vi "Dispose.vi"(8 "error in (no error)":errorcluster, 11 "PalmSens in":refnum<class "PalmSens.lvclass">) -> (0 "error out":errorcluster, 3 "PalmSens out":refnum<class "PalmSens.lvclass">)   [LabVIEW 2025, in "PalmSens.lvclass"]
uses:
  PalmSens.lvclass
  PalmSens.lvclass/PalmSens.ctl
  C:/Users/stef/code/palmsenssdk/labview/PalmSens/Libraries/PalmSens.Core.Simplified.LabVIEW.dll
  Libraries/PalmSens.Core.Simplified.LabVIEW.dll
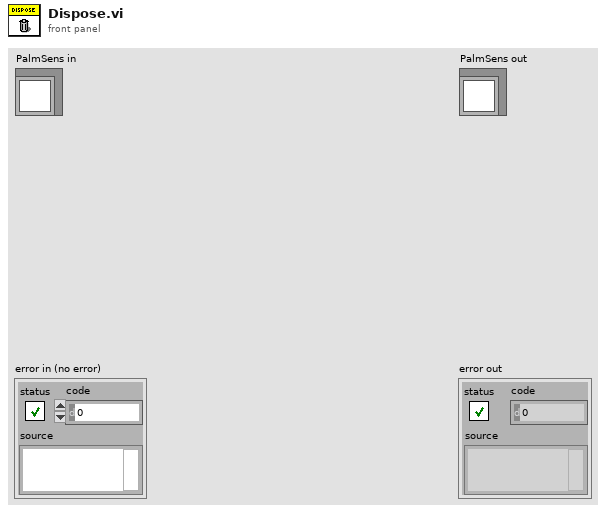
[diagram p1: front panel]
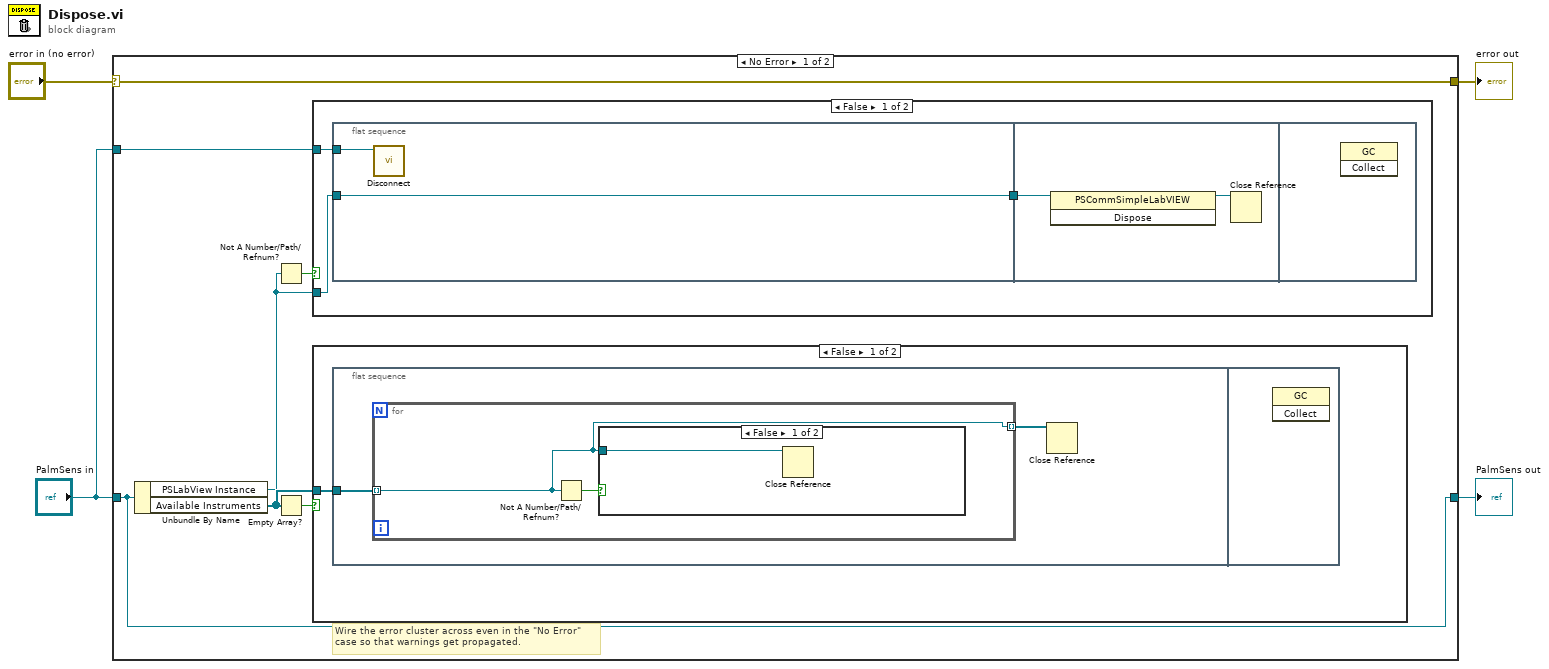
[diagram p0: block diagram]
diagram:
  n1 = case shown="No Error" "error in (no error)" {
    selector: "error in (no error)" -> [w11 w26]
    tunnel: [w11 w26] -> w3
    tunnel: [w10 w25] -> w2
    tunnel: "PalmSens in" -> [w10 w25]
    tunnel: "PalmSens in" -> [w5 _]
    frame No Error {
      # "Wire the error cluster across even in the \"No Error\"\ncase so that warnings get propagated."
      n2 = Unbundle By Name(w10) -> ("PSLabView Instance"=w6:refnum<k24>, "Available Instruments"=w8:refnum<k24>[])
      n3 = Not A Number/Path/Refnum?(number/path/refnum=w6) -> (NaN/Path/Refnum?=w7:bool)
      n4 = Empty Array?(array=w8) -> (empty?=w9:bool)
      n5 = case shown="False" w7 {
        tunnel: w6 -> [w14 _]
        tunnel: w5 -> [w12 _]
        frame False {
          n6 = flat-sequence {
            tunnel: w14 -> [w15]
            tunnel: [w15] -> w13
            tunnel: w12 -> [w16]
            tunnel: w13 -> [w18]
            frame #0 {
              n7 = call-dynamic "Disconnect.vi"("PalmSens in"=w16) -> ()  [unwired: 9 in, 2 out]
            }
            frame #1 {
              n8 = invoke class="PSCommSimpleLabVIEW" method="Dispose"(reference=w18) -> (reference out=w17:refnum<k24>)  [unwired: 2 in, 2 out]
              n9 = Close Reference(reference=w17) -> ()  [unwired: 1 in, 1 out]
            }
            frame #2 {
              n10 = invoke class="GC" method="Collect"() -> ()  [unwired: 3 in, 3 out]
            }
          }
        }
        frame True {
        }
      }
      n11 = case shown="False" w9 {
        tunnel: w8 -> [w19 _]
        frame False {
          n12 = flat-sequence {
            tunnel: w19 -> [w20]
            frame #0 {
              n13 = for {
                tunnel: w20 -> [w23] mode=indexing
                tunnel: [w23] -> w21 mode=indexing
                n14 = Not A Number/Path/Refnum?(number/path/refnum=w23) -> (NaN/Path/Refnum?=w22:bool)
                n15 = case shown="False" w22 {
                  tunnel: w23 -> [w24 _]
                  frame False {
                    n16 = Close Reference(reference=w24) -> ()  [unwired: 1 in, 1 out]
                  }
                  frame True {
                  }
                }
              }
              n17 = Close Reference(reference=w21) -> ()  [unwired: 1 in, 1 out]
            }
            frame #1 {
              n18 = invoke class="GC" method="Collect"() -> ()  [unwired: 3 in, 3 out]
            }
          }
        }
        frame True {
        }
      }
    }
    frame Error {
    }
  }
  "error out" <- w3
  "PalmSens out" <- w2
